vi "blokada wysylania manipulatora.vi"(6 "axis info":T1, 10 "wysylanie":bool) -> (0 "zakres Z":bool, 1 "zakres X":bool, 2 "blokadaa":bool, 3 "Wyslij":bool, 4 "zakres Y":bool, 5 "output cluster":T2)   [LabVIEW 2015]
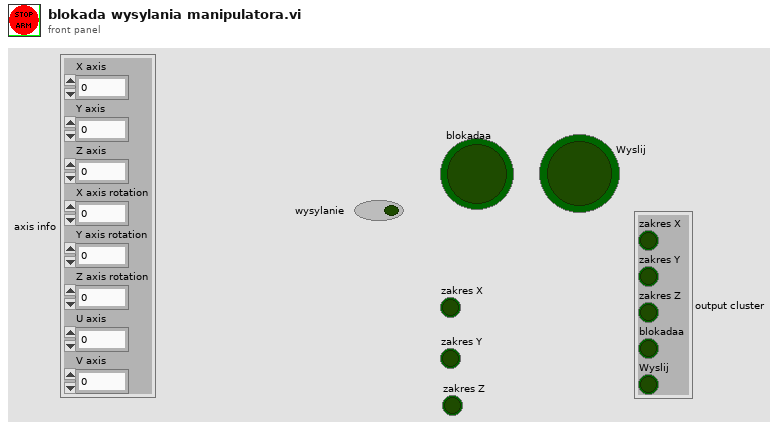
[diagram p1: front panel]
types:
  T1 = cluster{"X axis":i32, "Y axis":i32, "Z axis":i32, "X axis rotation":i32, "Y axis rotation":i32, "Z axis rotation":i32, "U axis":i32, "V axis":i32}
  T2 = cluster{"zakres X":bool, "zakres Y":bool, "zakres Z":bool, "blokadaa":bool, "Wyslij":bool}
  T3 = enum16{"Rising Edge", "Falling Edge", "Any Edge"}
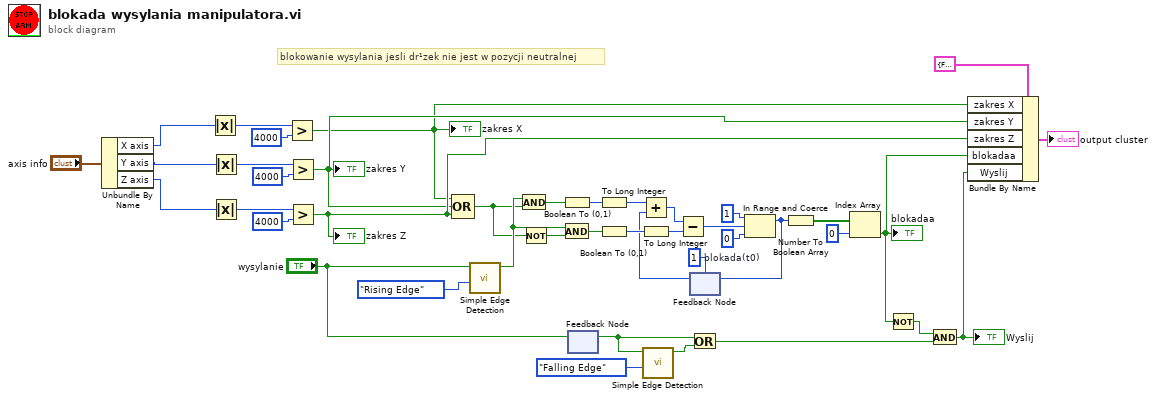
[diagram p0: block diagram]
diagram:
  w19 = 1  # blokada(t0)
  # "blokowanie wysylania jesli dr¹zek nie jest w pozycji neutralnej"
  n1 = Unbundle By Name("axis info") -> ("X axis"=w3:i32, "Y axis"=w2:i32, "Z axis"=w1:i32)
  n2 = Absolute Value(x=w3) -> (abs(x)=w28:i32)
  n3 = Absolute Value(x=w2) -> (abs(x)=w42:i32)
  n4 = Absolute Value(x=w1) -> (abs(x)=w26:i32)
  n5 = Greater?(x=w28, y=4000) -> (0:w6:bool)
  "zakres X" <- w6
  n6 = Greater?(x=w42, y=4000) -> (0:w7:bool)
  "zakres Y" <- w7
  n7 = Greater?(x=w26, y=4000) -> (0:w8:bool)
  "zakres Z" <- w8
  n8 = Compound Arithmetic op=OR(w6, w7, w8) -> (w18:bool)
  n9 = call "Simple Edge Detection.vi"("Mode"=T3."Rising Edge", "clk_in"="wysylanie") -> ("edge?"=w36:bool)  [unwired: 9 in]
  n10 = And(x=w36, y=w18) -> (x .and. y?=w31:bool)
  n11 = Not(x=w18) -> (.not. x?=w35:bool)
  n12 = Boolean To (0,1)(Boolean=w31) -> (0, 1=w24:i16)
  n13 = And(x=w36, y=w35) -> (x .and. y?=w34:bool)
  n14 = feedback #1() -> (w14:bool)  [unwired: 1 in]
  n15 = feedback-in #1("wysylanie") -> ()
  n16 = To Long Integer(number=w24) -> (32bit integer=w25:i32)
  n17 = Boolean To (0,1)(Boolean=w34) -> (0, 1=w22:i16)
  n18 = To Long Integer(number=w22) -> (32bit integer=w23:i32)
  n19 = call "Simple Edge Detection.vi"("Mode"=T3."Falling Edge", "clk_in"=w14) -> ("edge?"=w13:bool)  [unwired: 9 in]
  n20 = feedback #2(w19) -> (w21:i32)
  n21 = Add(x=w25, y=w21) -> (x+y=w38:i32)
  n22 = Subtract(x=w38, y=w23) -> (x-y=w37:i32)
  n23 = Or(x=w14, y=w13) -> (x .or. y?=w12:bool)
  n24 = In Range and Coerce(upper limit=1 ("lower limit"), x=w37, lower limit=0) -> (coerced(x)=w20:i32)  [unwired: 1 out]
  n25 = feedback-in #2(w20) -> ()
  n26 = Number To Boolean Array(number=w20) -> (Boolean array=w39:bool[])
  n27 = Index Array(array=w39, index=0) -> (element=w9:bool)
  "blokadaa" <- w9
  n28 = Not(x=w9) -> (.not. x?=w16:bool)
  n29 = And(x=w16, y=w12) -> (x .and. y?=w10:bool)
  "Wyslij" <- w10
  n30 = Bundle By Name(cluster=T2 {"zakres X"=FALSE, "zakres Y"=FALSE, "zakres Z"=FALSE, "blokadaa"=FALSE, "Wyslij"=FALSE} ("Cluster"), "zakres X"=w6, "zakres Y"=w7, "zakres Z"=w8, "blokadaa"=w9, "Wyslij"=w10) -> (→"output cluster":T2)
